vi "take piece from floor.vi"(10 "y":dbl, 11 "m":i32) -> ()   [LabVIEW 2018]
panel:
  in  "speed":dbl
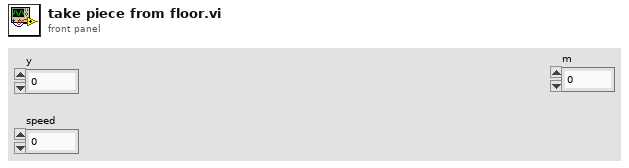
[diagram p1: front panel]
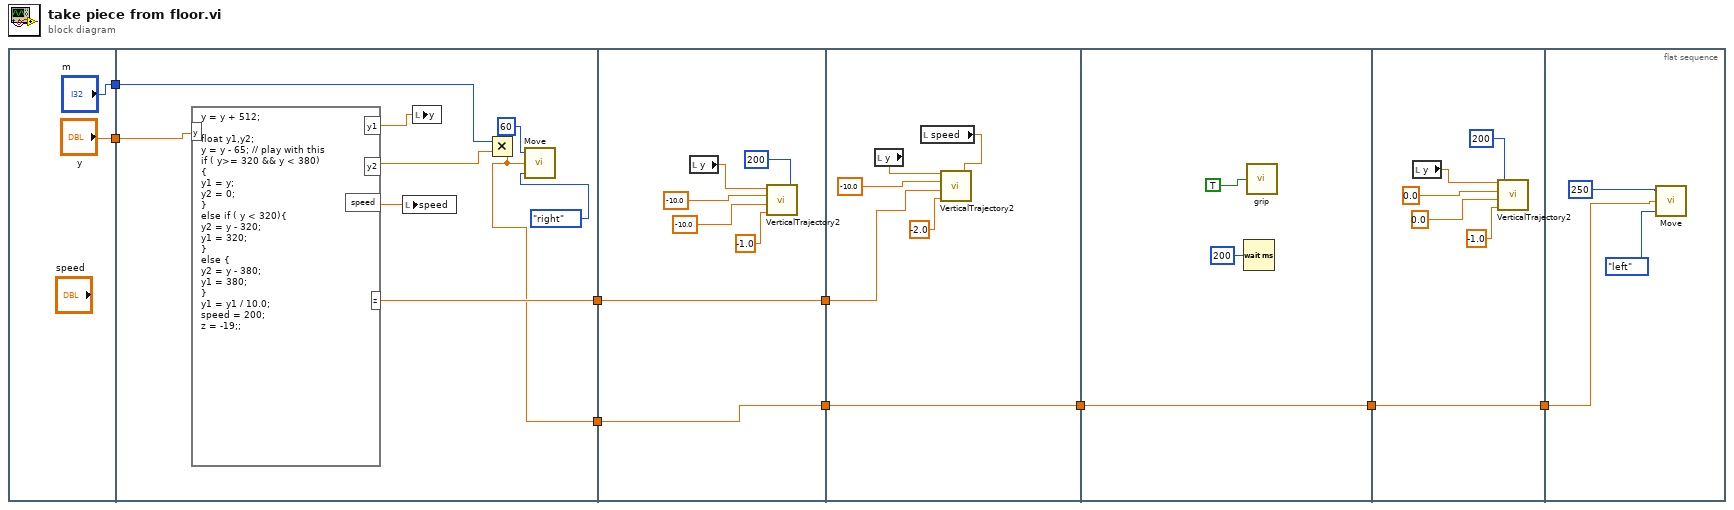
[diagram p0: block diagram]
diagram:
  n1 = flat-sequence {
    tunnel: ["y"] -> w9
    tunnel: ["m"] -> w1
    tunnel: w9 -> [w17]
    tunnel: [w16] -> w8
    tunnel: [w13] -> w6
    tunnel: w1 -> [w12]
    tunnel: [w22] -> w7
    tunnel: w8 -> [w22]
    tunnel: w6 -> [w21]
    tunnel: [w21] -> w5
    tunnel: w7 -> [w29]
    tunnel: w5 -> [w28]
    tunnel: [w28] -> w4
    tunnel: w4 -> [w34]
    tunnel: [w34] -> w3
    tunnel: w3 -> [w37]
    tunnel: [w37] -> w2
    tunnel: w2 -> [w44]
    frame #0 {
    }
    frame #1 {
      n2 = formula code="y = y + 512;\n\nfloat y1,y2;\ny = y - 65; // play with this \nif ( y>= 320 && y < 380)\n{\ny1 = y;\ny2 = 0;\n}\nelse if ( y < 320){\ny2 = y - 320;\ny1 = 320;\n}\nelse {\ny2 = y - 380;\ny1 = 380;\n}\ny1 = y1 / 10.0;\nspeed = 200;\nz = -19;;"("y"=w17) -> ("y1"=w19:dbl, "y2"=w14:dbl, "speed"=w20:dbl, "z"=w16:dbl)
      n3 = local write "speed"(w20) -> ()
      n4 = local write "y"(w19) -> ()
      n5 = Multiply(x=w12, y=w14) -> (x*y=w13:dbl)
      n6 = call "Move.vi"("Enum"=enum16{"forward", "backward", "left", "right"}."right", "distance"=w13, "speed"=60) -> ()  [unwired: 1 in]
    }
    frame #2 {
      n7 = local read "y"() -> (w24:dbl)
      n8 = call "VerticalTrajectory2.vi"("speed 1"=200, "step"=-1.0, "z2"=-10.0, "z1"=-10.0, "x"=w24) -> ()  [unwired: 3 in]
    }
    frame #3 {
      n9 = local read "y"() -> (w33:dbl)
      n10 = local read "speed"() -> (w30:dbl)
      n11 = call "VerticalTrajectory2.vi"("speed 1"=w30, "step"=-2.0, "z2"=w29, "z1"=-10.0, "x"=w33) -> ()  [unwired: 3 in]
    }
    frame #4 {
      n12 = Wait (ms)(milliseconds to wait=u32 200) -> ()  [unwired: 1 out]
      n13 = call "grip.vi"("grip"=TRUE) -> ()
    }
    frame #5 {
      n14 = local read "y"() -> (w39:dbl)
      n15 = call "VerticalTrajectory2.vi"("speed 1"=200, "step"=-1.0, "z2"=0.0, "z1"=0.0, "x"=w39) -> ()  [unwired: 3 in]
    }
    frame #6 {
      n16 = call "Move.vi"("Enum"=enum16{"forward", "backward", "left", "right"}."left", "distance"=w44, "speed"=250) -> ()  [unwired: 1 in]
    }
  }
